vi "Init.vi"(4 "error in":errorcluster) -> (0 "error out":errorcluster, 1 "DAQ":bool, 2 "Device Connection Cluster":T1, 3 "Servo":bool)   [LabVIEW 2013]
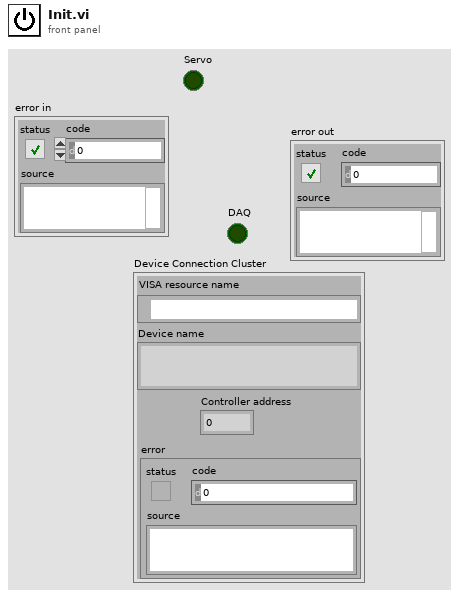
[diagram p1: front panel]
types:
  T1 = cluster{"VISA resource name":refnum<visa-resource-name>, "Device name":string, "Controller address":i32, "error":errorcluster}
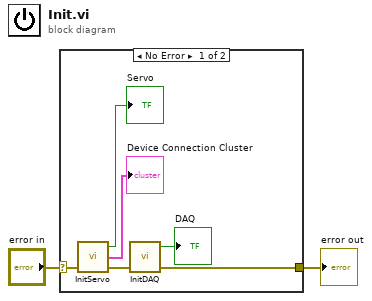
[diagram p0: block diagram]
diagram:
  n1 = case shown="No Error" "error in" {
    selector: "error in" -> [w6 w9]
    tunnel: [w4 w9] -> w2
    frame No Error {
      n2 = call "InitServo.vi"("error in"=w6) -> ("error out"=w5:errorcluster, "Device Connection Cluster"=→"Device Connection Cluster":T1, "Boolean"=→"Servo":bool)  [unwired: 2 in]
      n3 = call "InitDAQ.vi"("error in"=w5) -> ("error out"=w4:errorcluster, "DAQ connected?"=→"DAQ":bool)  [unwired: 3 in]
    }
    frame Error {
    }
  }
  "error out" <- w2
